vi "Main根目录.vi"() -> ()   [LabVIEW 2013]
panel:
  in  "Main根目录":path
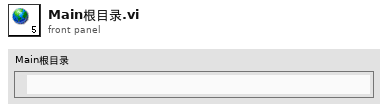
[diagram p1: front panel]
diagram:
